vi "Initialize TreeBrowserWF.vi"(8 "error in (no error)":errorcluster, 9 "Refs":T1[](array[typedef]) format="%.0x", 10 "Node Pointer":T2, 11 "TreeBrowserRef":refnum<k24>) -> (0 "error out":errorcluster, 2 "Channels":variant, 3 "TreeBrowserRef 2":refnum<k24>)   [LabVIEW 2013, in "OPC UA Client System Explorer.lvlib"]
uses:
  OPC UA Client System Explorer.lvlib
  <vilib>/NI Veristand/Custom Device API/Custom Device Pointer.ctl
  NationalInstruments.VeriStand.SystemStorage
  NationalInstruments.VeriStand.SystemStorageUI
  <vilib>/NI Veristand/Custom Device API/Custom Device Item Ref.ctl
  NationalInstruments.VeriStand
  <vilib>/NI Veristand/Custom Device API/Custom Device API.lvlib
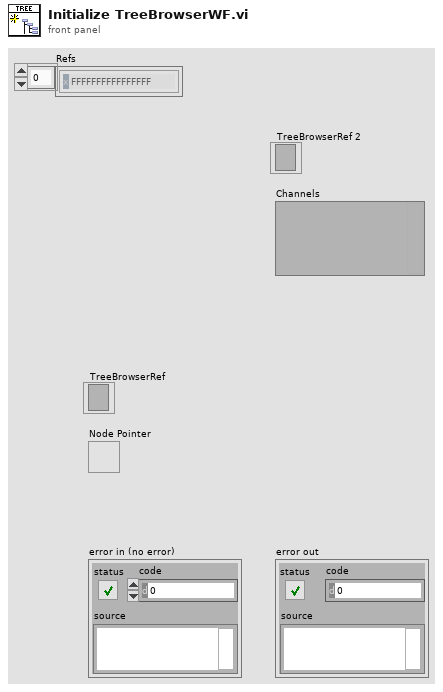
[diagram p1: front panel]
types:
  T1 = typedef "Custom Device API.lvlib/Custom Device Item Ref.ctl" = u64
  T2 = typedef "Custom Device API.lvlib/Custom Device Pointer.ctl" = refnum<k24>
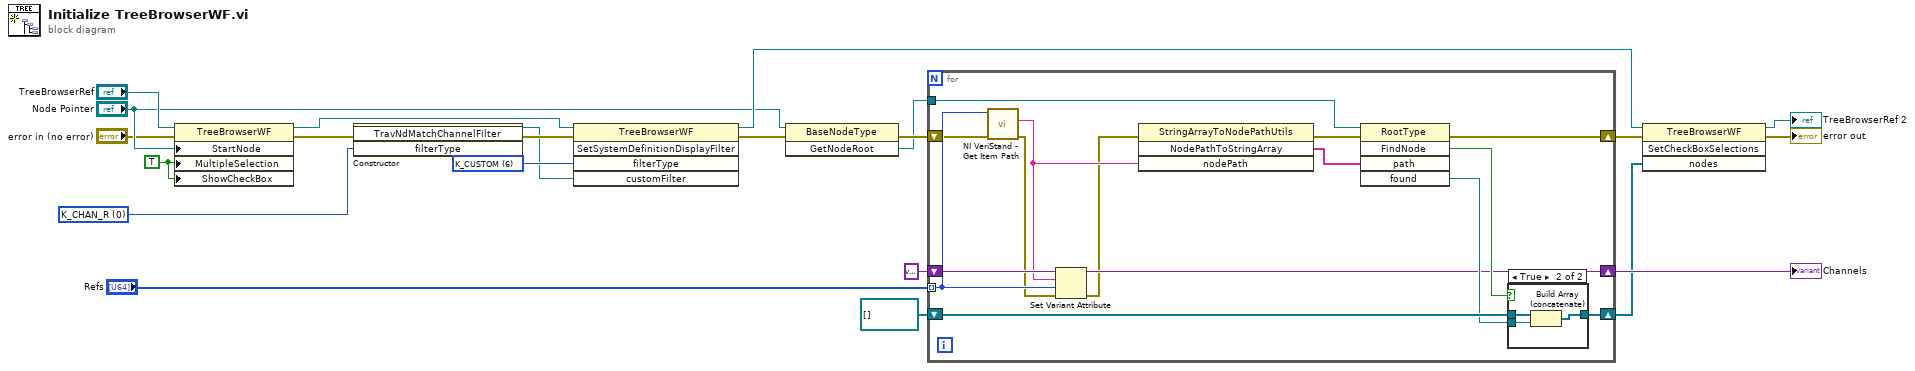
[diagram p0: block diagram]
diagram:
  w7 = u8 0 items=["K_CHAN_R", "K_CHAN_W", "K_CHAN_VOLT", "K_CHAN_FAULT"] ("filterType")
  w16 = TRUE ("MultipleSelection")
  w8 = u8 6 items=["K_CHAN_R", "K_CHAN_W", "K_CHAN_RW", "K_CHAN_VOLT", "K_CHAN_FAULT", "K_ALL", "K_CUSTOM", "K_CHAN_R_VIS", "K_CHAN_W_VIS", "K_CHAN_RW_VIS", "K_CHAN_VOLT_VIS", "K_CHAN_FAULT_VIS", "K_WAVE", "K_WAVE_VIS", "K_WAVE_DBL", "K_WAVE_CDB", "K_WAVE_DBL_VIS", "K_WAVE_CDB_VIS"] ("filterType")
  n1 = property class="TreeBrowserWF"(reference="TreeBrowserRef", error in="error in (no error)", "StartNode"="Node Pointer", "MultipleSelection"=w16, "ShowCheckBox"=w16) -> (reference out=w10:refnum<k24>, error out=w3:errorcluster)
  n2 = constructor class="TravNdMatchChannelFilter"(error in=w3, "filterType"=w7) -> (reference out=w1:refnum<k24>, error out=w2:errorcluster)  [unwired: 2 in, 2 out]
  n3 = invoke class="TreeBrowserWF" method="SetSystemDefinitionDisplayFilter"(reference=w10, error in=w2, "filterType"=w8, "customFilter"=w1) -> (reference out=w12:refnum<k24>, error out=w21:errorcluster)  [unwired: 1 in, 3 out]
  n4 = invoke class="BaseNodeType" method="GetNodeRoot"(reference="Node Pointer", error in=w21) -> (error out=w22:errorcluster, "GetNodeRoot"=w20:refnum<k24>)  [unwired: 1 in, 1 out]
  n5 = for {
    shift-right: [w34] -> w15
    shift-left: w22 -> [w26]
    tunnel: "Refs" -> [w27] mode=indexing
    tunnel: w20 -> [w37]
    shift-right: [w31] -> w17
    shift-left: refnum<k24>[] [] -> [w32]
    shift-right: [w28] -> w19
    shift-left: variant -> [w29]
    n6 = call <vilib>:"NI VeriStand - Get Item Path.vi"("error in (no error)"=w26, "Item Ref in"=w27) -> ("error out"=w24:errorcluster, "Path"=w25:string)  [unwired: 6 in, 2 out]
    n7 = Set Variant Attribute(Variant=w29, name=w25, value=w27, error in=w24) -> (Variant out=w28:variant, error out=w23:errorcluster)  [unwired: 1 out]
    n8 = invoke class="StringArrayToNodePathUtils" method="NodePathToStringArray"(error in=w23, "nodePath"=w25) -> (error out=w35:errorcluster, "NodePathToStringArray"=w36:string[])  [unwired: 2 in, 2 out]
    n9 = invoke class="RootType" method="FindNode"(reference=w37, error in=w35, "path"=w36) -> (error out=w34:errorcluster, "FindNode"=w33:bool, "found"=w30:refnum<k24>)  [unwired: 2 in, 2 out]
    n10 = case shown="True" w33 {
      tunnel: w32 -> [w38 w41]
      tunnel: [w38 w39] -> w31
      tunnel: w30 -> [_ w40]
      frame False {
      }
      frame True {
        n11 = Build Array (concatenate)(w41, w40) -> (w39:refnum<k24>[])
      }
    }
  }
  "Channels" <- w19
  n12 = invoke class="TreeBrowserWF" method="SetCheckBoxSelections"(reference=w12, error in=w15, "nodes"=w17) -> (reference out=→"TreeBrowserRef 2":refnum<k24>, error out=→"error out":errorcluster)  [unwired: 1 in, 2 out]
